vi "Forward Pass (AutoEncoder).vi"(0 "x":dbl[](array[numeric])=[0.0, 0.1111111111111111, 0.2222222222222222, 0.3333333333333333, 1.0, 0.8888888888888888, 0.7777777777777778, 0.6666666666666666], 1 "Wxh":dbl[][](array[numeric])=[[0.21505248184279538, 1.3189727439634347, 0.48891156267063407, 0.46110723166267786, -2.894692829733287, -1.8460923219121097, -1.8192019685340954, -0.5062553613618253], [1.6209332090971538, -1.7971354604553609, 1.6200200442111778, 2.363410811791121, 3.9919249354601822, 3.222634360023979, 3.322833501710172, 1.931809225857201], [1.1823589897829023, -1.8436896029229477, -0.9434139364780342, -0.10498125402967093, 1.0402991449686243, 0.7474478164291856, 1.7367285875359595, 0.7135503045205506], [0.7631971643466479, -1.4265164161917685, 0.7911698629363837, 2.23794677103215, -1.3092600566257102, -0.04354306266684625, -1.1164324621878867, -0.37441280081456096]], 2 "by":dbl[](array[numeric])=[-0.02963272382849274, -0.04802494337274095, 1.661658647173072, -0.3071258628271679, 1.4859107856525422, -0.8125993201472581, -0.21904939732707582, 1.338412698345055], 3 "Wh,xhat":dbl[][](array[numeric])=[[0.3163826991063027, 0.6928663099716998, 0.59602455786111, 0.946061549540873], [0.39285570927746805, -1.5385544459498817, 1.9611797116439431, -0.13028708690539617], [0.6675621606400596, -1.0746724587343237, -0.5330674970736385, -0.8386692340280304], [-0.6412693821172979, -1.2242259554716968, 2.220729576282102, 1.0002800297160181], [0.042438249888928005, -1.105442738544762, 1.259696385782826, 0.5995300586910652], [-0.15650534879719294, -0.20835889099398353, 0.0015925026592361056, -1.7579270043774835], [-1.1099322243336174, 0.8446263194639312, 0.08102757284525873, 1.042377326793812], [0.6656770307122334, -0.4868273812531405, 2.026427876951232, 1.550642598683917]], 4 "bh":dbl[](array[numeric])=[0.14338102802404934, -1.6903645688894957, 1.4317151302429396, -1.4688435828569493]) -> (14 "y":dbl[](array[numeric]), 15 "tanh(y)":dbl[](array[numeric]), 16 "x_hat":dbl[](array[numeric])=[-4.85722573273506e-17, 0.11111111111111081, 0.22222222222221744, 0.3333333333333306, 0.9999999999999998, 0.8888888888888888, 0.7777777777777778, 0.6666666666666639], 18 "error":dbl[](array[numeric]))   [LabVIEW 2014]
uses:
  <vilib>/Analysis/baseanly.llb/A x Vector.vi
  <vilib>/Analysis/NI_AALBase.lvlib
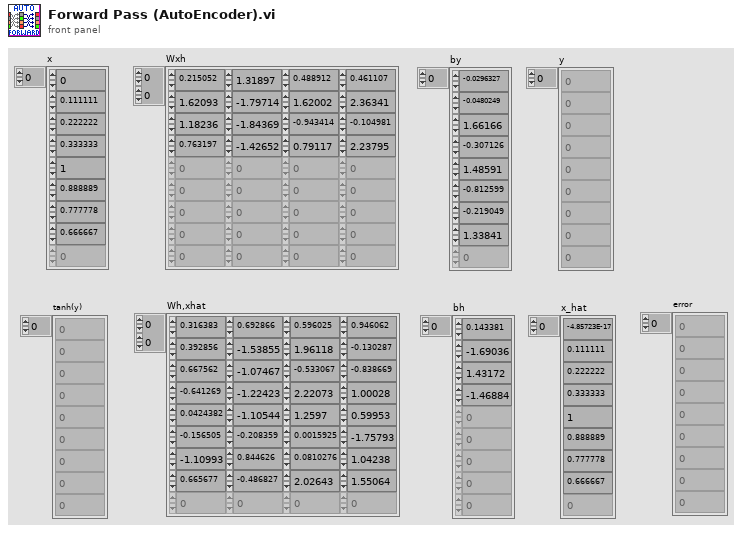
[diagram p1: front panel]
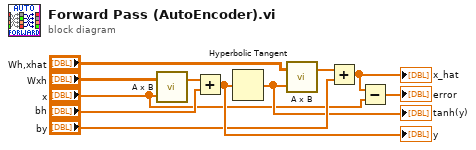
[diagram p0: block diagram]
diagram:
  n1 = call-poly <vilib>:"A x B.vi"("Vector"="x", "A"="Wxh") -> ("A x Vector"=w10:dbl[])  [unwired: 1 out]
  n2 = Add ("Add.vi")(x=w10, y="bh") -> (x+y=w8:dbl[])
  "y" <- w8
  n3 = Hyperbolic Tangent(1:w8) -> (0:w5:dbl[])
  "tanh(y)" <- w5
  n4 = call-poly <vilib>:"A x B.vi"("Vector"=w5, "A"="Wh,xhat") -> ("A x Vector"=w4:dbl[])  [unwired: 1 out]
  n5 = Add ("Add.vi")(x=w4, y="by") -> (x+y=w3:dbl[])
  "x_hat" <- w3
  n6 = Subtract(x=w3, y="x") -> (x-y=→"error":dbl[])
